vi "Initialize Session with NVMEM Areas.vi"(0 "NVMEM areas":refnum<k21>, 7 "reservation access (Read/Write)":i32(ring)=3 items=["None"=0, "Read Only"=1, "Read/Write"=3], 9 "reservation group":string, 11 "error in (no error)":errorcluster, 12 "connect timeout (60 sec)":dbl=60.0, 13 "reservation timeout (0 sec)":dbl) -> (4 "session out":refnum<k21>, 15 "error out":errorcluster)   [LabVIEW 2020, in "SLSC.lvlib"]
doc: "Initializes an SLSC session with one or multiple NVMEM areas. The session opens network connections for NVMEM areas. If <B>reservation access</B> is set to <B>Read Only</B> or <B>Read/Write</B>, the session also reserves the devices."
uses:
  <vilib>/SLSC/SLSC.lvlib
  nislsclvapi.dll
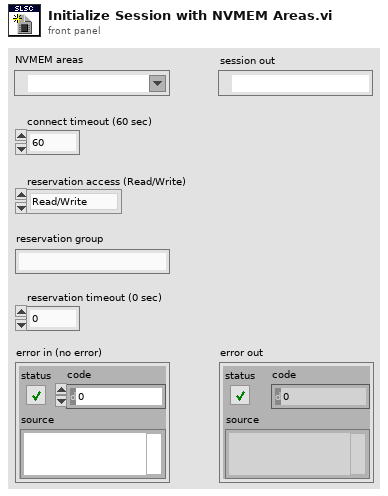
[diagram p1: front panel]
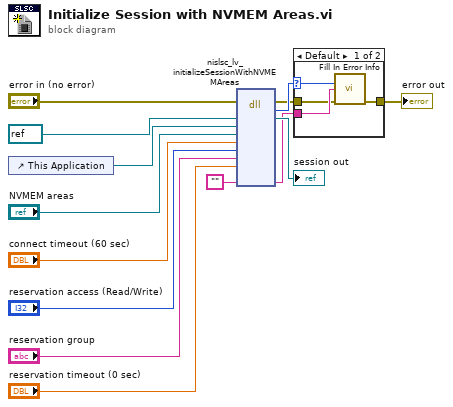
[diagram p0: block diagram]
diagram:
  n1 = control-ref of="This Application"() -> (w6:refnum<vi>)
  n2 = dll-call lib="nislsclvapi.*" fn="nislsc_lv_initializeSessionWithNVMEMAreas"(error in="error in (no error)", "session"=refnum<k21> refnum ("SLSC Session"), "lvAppRef"=w6, "nvmemAreas"="NVMEM areas", "connectTimeout"="connect timeout (60 sec)", "reservationAccess"="reservation access (Read/Write)", "reservationGroup"="reservation group", "reservationTimeout"="reservation timeout (0 sec)", "extendedErrorInfo"="") -> (error out=w8:errorcluster, "return type"=w10:i32, "session"=→"session out":refnum<k21>, "extendedErrorInfo"=w9:string)  [unwired: 10 in, 1 out]
  n3 = case shown="Default" w10 {
    selector: w10 -> [w18 _]
    tunnel: w9 -> [w17 _]
    tunnel: w8 -> [w16 w19]
    tunnel: [w15 w19] -> w7
    frame Default {
      n4 = call <vilib>:"Fill In Error Info.vi"("status code"=w18, "extended error info"=w17, "error in"=w16) -> ("error out"=w15:errorcluster)  [unwired: 12 in]
    }
    frame 0 {
    }
  }
  "error out" <- w7
